vi "AddNode.vi"(5 "UID":i32, 9 "VI_AST in":refnum<class "VI_AST.lvclass">) -> (3 "VI_AST out":refnum<class "VI_AST.lvclass">, 4 "index":i32)   [LabVIEW 2014, in "Raspberry Pi Compatible Compiler for LabVIEW.lvlib" / "VI_AST.lvclass"]
uses:
  VI_AST.lvclass
  VI_AST.lvclass/VI_AST.ctl
  DAG/DAG/DAG.lvclass
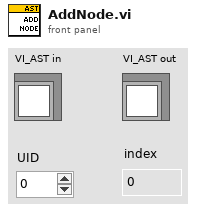
[diagram p1: front panel]
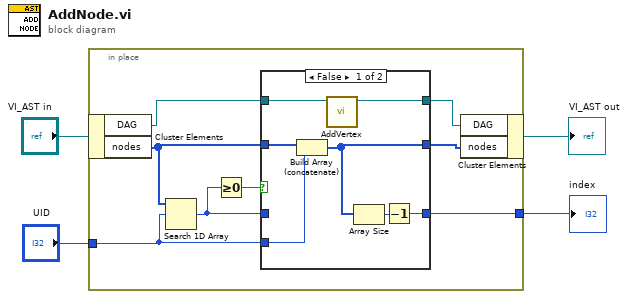
[diagram p0: block diagram]
diagram:
  n1 = in-place {
    in-place-border: "UID" -> [w9]
    in-place-border: [w8] -> w1
    n2 = in-place-cluster #1("VI_AST in") -> ("DAG"=w6:refnum<class "DAG.lvclass">, "nodes"=w11:i32[])
    n3 = Search 1D Array(1D array=w11, element=w9) -> (index of element=w7:i32)  [unwired: 1 in]
    n4 = Greater Or Equal To 0?(x=w7) -> (x >= 0?=w12:bool)
    n5 = case shown="False" w12 {
      tunnel: w11 -> [w19 w22]
      tunnel: [w17 w22] -> w10
      tunnel: w9 -> [w18 _]
      tunnel: [w13 w21] -> w8
      tunnel: w7 -> [_ w21]
      tunnel: w6 -> [w15 w20]
      tunnel: [w14 w20] -> w5
      frame False {
        n6 = Build Array (concatenate)(w19, w18) -> (w17:i32[])
        n7 = call "AddVertex.vi"("DAG in"=w15) -> ("DAG out"=w14:refnum<class "DAG.lvclass">)  [unwired: 7 in, 1 out]
        n8 = Array Size(array=w17) -> (size(s)=w16:i32)
        n9 = Decrement(x=w16) -> (x-1=w13:i32)
      }
      frame True {
      }
    }
    n10 = in-place-cluster #1("DAG"=w5, "nodes"=w10) -> (→"VI_AST out":refnum<class "VI_AST.lvclass">)
  }
  "index" <- w1
